vi "Main.vi"(11 "Module Admin":refnum<class "Delacor_lib_QMH_Module Admin.lvclass">) -> ()   [LabVIEW 2019, in "CONEXIÓN CON EL MICRO.lvlib"]
doc: "This template is based off of the Queued Message Handler design pattern and the Queued Message Handler project template that ships with LabVIEW.\n\nThe main difference is that the queue is private to this module and communication between modules is performed via Broadcast and Request events.\n\nRequest events are wrapped in public API methods and are handled in the Event Handling Loop (EHL) of this VI. Any module can register for Broadcast events sent by this module. The EHL generates messages based on user interface actions.\n\nThe Message Handling Loop (MHL) processes messages generated by the EHL, or by other messages. The messages are string values, so new messages can be added easily to the Message Cases case structure in the MHL. Each message cluster can also provide an optional value for Message Data, which is a variant that can be converted to whatever message-specific data is required.\n_____\nBased on Delacor QMH Project Template 5.0.0.82."
uses:
  <vilib>/Delacor/Delacor QMH/Libraries/Module Admin_class/Delacor_lib_QMH_Module Admin.lvclass
  Module Data--cluster.ctl
  <vilib>/Delacor/Delacor QMH/Libraries/Message Queue_class/Delacor_lib_QMH_Message Queue.lvclass/Delacor_lib_QMH_Message Queue.ctl
  Stop Argument--cluster.ctl
  <vilib>/Delacor/Delacor QMH/Libraries/Module Admin_class/Delacor_lib_QMH_Module Admin.lvclass/Delacor_lib_QMH_Module Admin.ctl
  START HELPER LOOP Argument--cluster.ctl
  STOP HELPER LOOP Argument--cluster.ctl
  <vilib>/Utility/miscctls.llb/LVPointTypeDef.ctl
  <vilib>/Delacor/Delacor QMH/Libraries/Message Queue_class/Delacor_lib_QMH_Enqueue Message (Single).vi
  <vilib>/Delacor/Delacor QMH/Libraries/Module Admin_class/Delacor_lib_QMH_Get External Launch.vi
  <vilib>/Utility/error.llb/Error Cluster From Error Code.vi
  <vilib>/ErrorRing/Error Ring.xnode
  <vilib>/Delacor/Delacor QMH/Libraries/Message Queue_class/Delacor_lib_QMH_Message Queue.lvclass
panel:
  in  "Simulate MHL Error":bool
  in  "Simulate EHL Error":bool
  out "error out":errorcluster
  out "Status":string
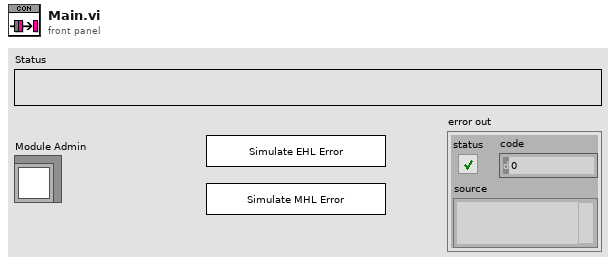
[diagram p1: front panel]
types:
  T1 = typedef "CONEXIÓN CON EL MICRO.lvlib/Request Events--cluster.ctl" = cluster{"Stop Module":refnum<user-event>, "Show Panel":refnum<user-event>, "Hide Panel":refnum<user-event>, "Get Module Execution Status":refnum<user-event>, "Show Diagram":refnum<user-event>, "START HELPER LOOP":refnum<user-event>, "STOP HELPER LOOP":refnum<user-event>}
  T2 = typedef "CONEXIÓN CON EL MICRO.lvlib/Module Data--cluster.ctl" = cluster{"Status":string}
  T3 = enum32{"invalid lock state", "Not Locked", "Locked (No Password)", "Password-protected"}
  T4 = typedef "CONEXIÓN CON EL MICRO.lvlib/Stop Argument--cluster.ctl" = cluster{"Origin":string, "Exit via Stop Module Req?":bool, "Wait for Module to stop?":bool}
  T5 = typedef "CONEXIÓN CON EL MICRO.lvlib/START HELPER LOOP Argument--cluster.ctl" = cluster{"DELAY TIMEOUT":i32}
  T6 = typedef "CONEXIÓN CON EL MICRO.lvlib/STOP HELPER LOOP Argument--cluster.ctl" = cluster{"Boolean":bool}
  T7 = typedef "LVPointTypeDef.ctl" = cluster{"Horizontal":i16, "Vertical":i16}
  T8 = enum32{"Invalid", "Standard", "Closed", "Hidden", "Minimized", "Maximized"}
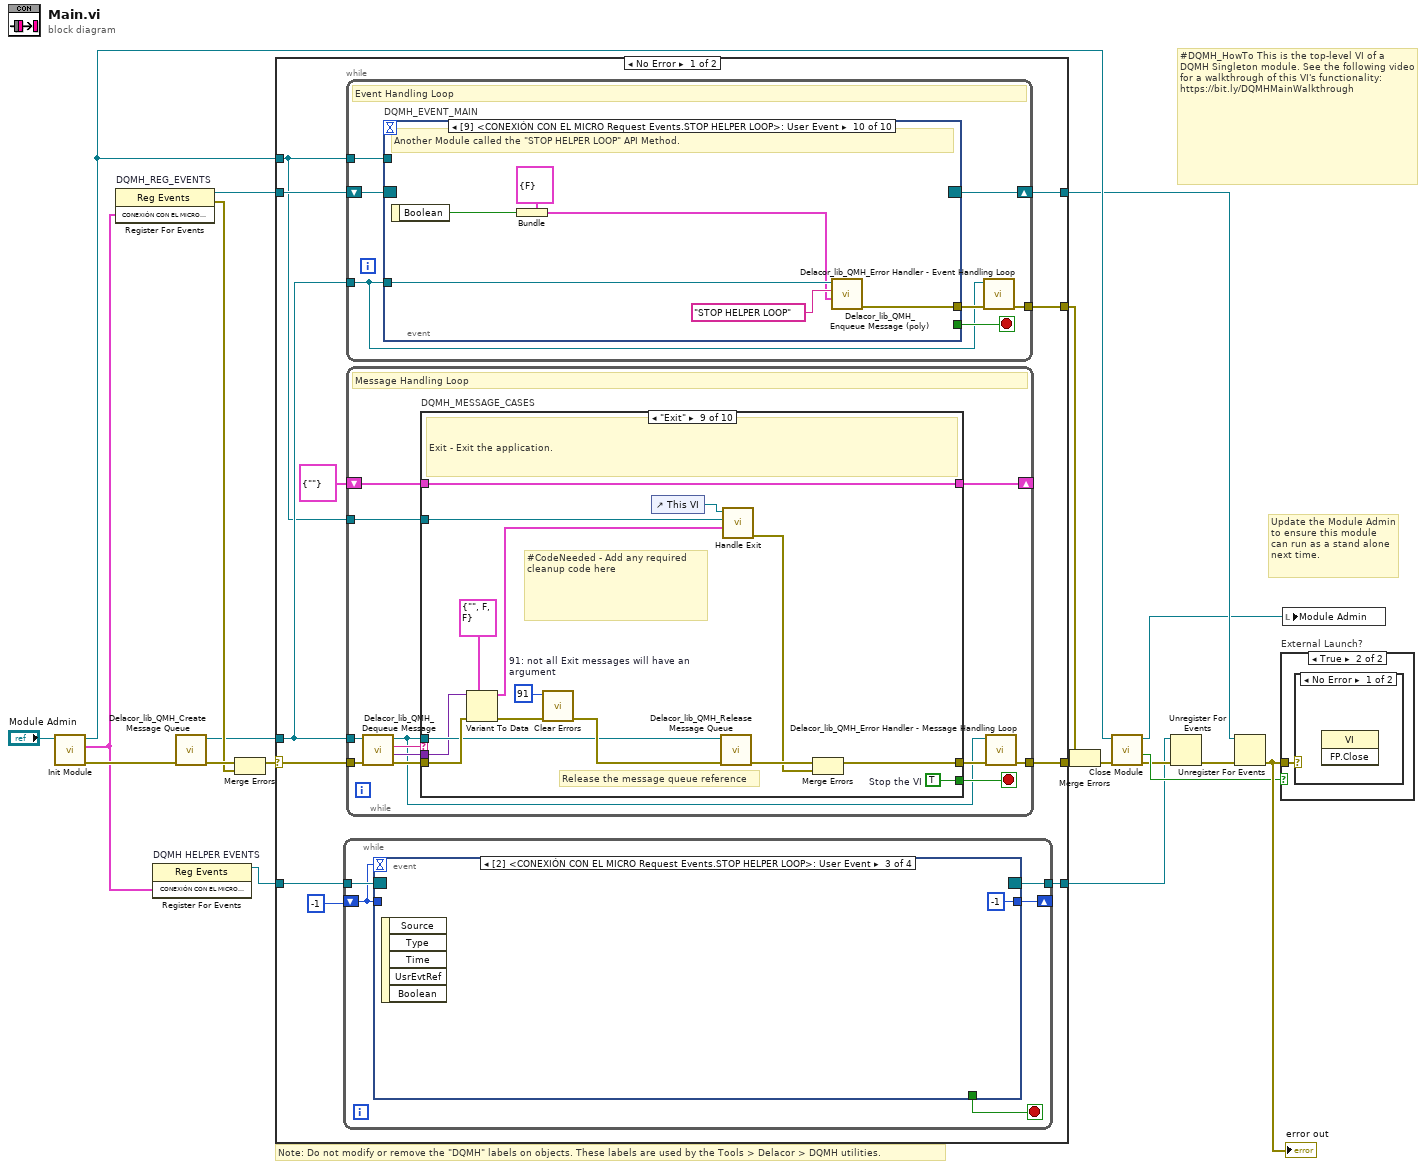
[diagram p0: block diagram]
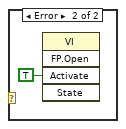
[diagram p3: hidden frame]
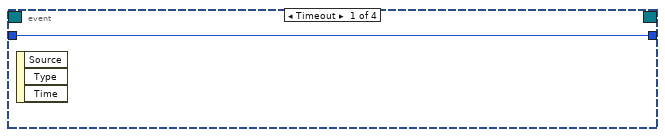
[diagram p4: hidden frame]
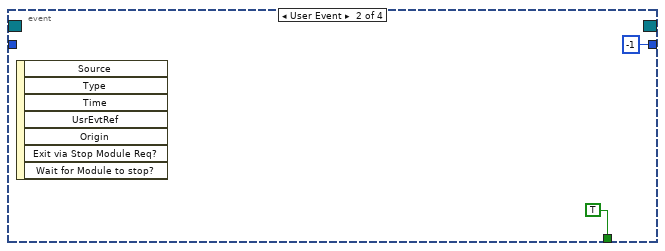
[diagram p5: hidden frame]
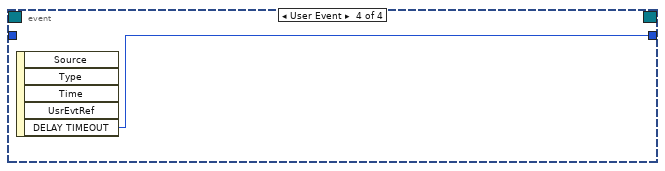
[diagram p6: hidden frame]
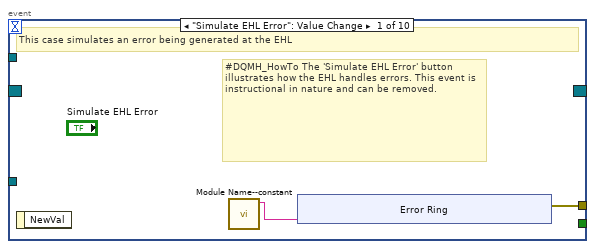
[diagram p7: hidden frame]
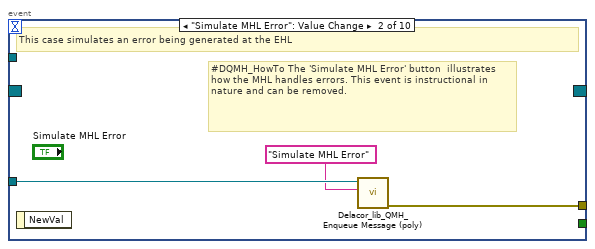
[diagram p8: hidden frame]
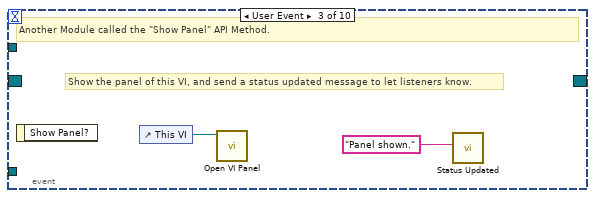
[diagram p9: hidden frame]
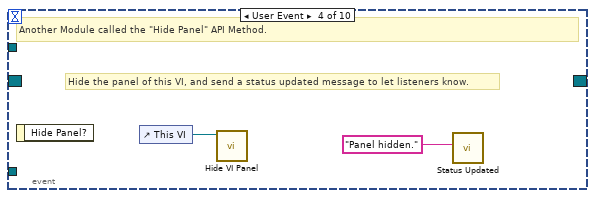
[diagram p10: hidden frame]
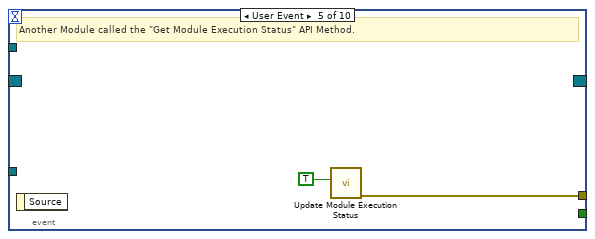
[diagram p11: hidden frame]
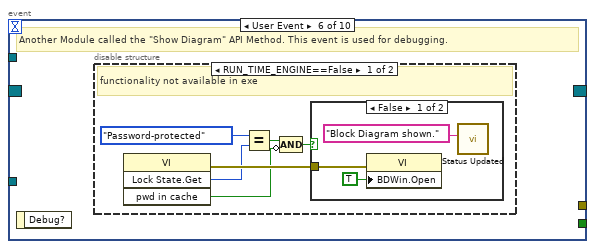
[diagram p12: hidden frame]
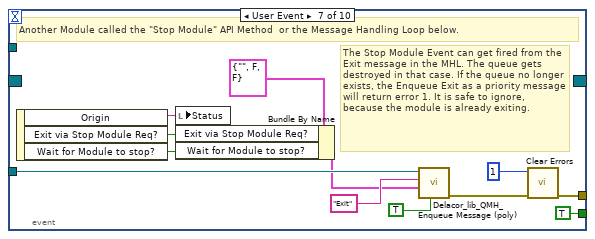
[diagram p15: hidden frame]
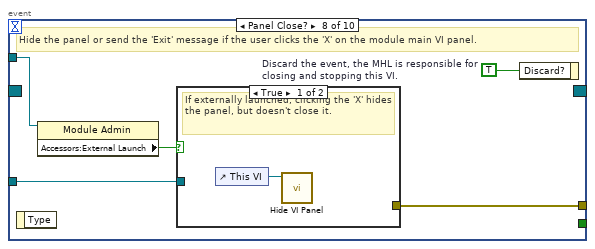
[diagram p16: hidden frame]
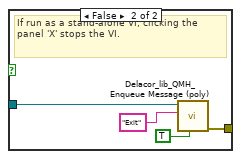
[diagram p17: hidden frame]
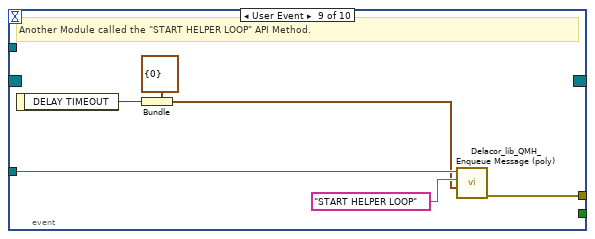
[diagram p18: hidden frame]
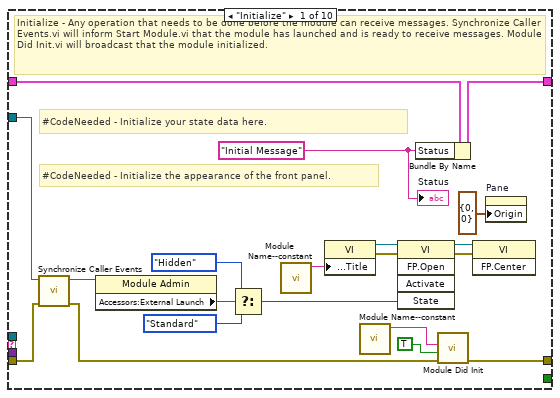
[diagram p19: hidden frame]
diagram:
  # "#DQMH_HowTo This is the top-level VI of a DQMH Singleton module. See the following video for a walkthrough of this VI's functionality: https://bit.ly/DQMHMainWalkthrough"
  # "Note: Do not modify or remove the \"DQMH\" labels on objects. These labels are used by the Tools > Delacor > DQMH utilities."
  # "Update the Module Admin to ensure this module can run as a stand alone next time."
  n1 = call "Init Module.vi"("Singleton Module Admin in"="Module Admin") -> ("error out"=w19:errorcluster, "CONEXIÓN CON EL MICRO Request Events"=w2:T1, "Singleton Module Admin out"=w12:refnum<class "Delacor_lib_QMH_Module Admin.lvclass">)  [unwired: 8 in]
  n2 = register-events "DQMH_REG_EVENTS"(w2) -> (reference out=w10:refnum<event-registration>, error out=w13:errorcluster)  [unwired: 2 in]
  n3 = register-events "DQMH HELPER EVENTS"(w2) -> (reference out=w1:refnum<event-registration>)  [unwired: 2 in, 1 out]
  n4 = call <vilib>:"Delacor_lib_QMH_Create Message Queue.vi"("error in (no error)"=w19) -> ("error out"=w15:errorcluster, "Message Queue"=w9:refnum<class "Delacor_lib_QMH_Message Queue.lvclass">)  [unwired: 9 in]
  n5 = Merge Errors(w15, w13) -> (w14:errorcluster)
  n6 = case shown="No Error" w14 {
    selector: w14 -> [w29 w222]
    tunnel: [w31 w221] -> w20
    tunnel: [w28 w227] -> w11
    tunnel: w10 -> [w26 w227]
    tunnel: w9 -> [w25 w220]
    tunnel: [w30 _] -> w18
    tunnel: w12 -> [w24 w223]
    tunnel: [w23 w219] -> w3
    tunnel: w1 -> [w22 w219]
    frame No Error {
      n7 = while {
        tunnel: [w36] -> w23
        tunnel: w22 -> [w35]
        shift-right: [w34] -> _
        shift-left: -1 -> [w33]
        stop <- w32 stop-if-true
        n8 = event shown="[2] <CONEXIÓN CON EL MICRO Request Events.STOP HELPER LOOP>: User Event" {
          selector: w35 -> [_ _ _ _]
          dyn-events: [_ _ _ _] -> w36
          timeout: w33 -> [_ _ _ _]
          tunnel: [w37 -1 ("DELAY TIMEOUT") -1 ("DELAY TIMEOUT") w41] -> w34
          tunnel: w33 -> [w37 _ _ _]
          tunnel: [_ TRUE _ _] -> w32
          event Timeout {
            n9 = event-data() -> ()  [unwired: 1 in, 3 out]
          }
          event User Event {
            n10 = event-data() -> ()  [unwired: 1 in, 7 out]
          }
          event User Event {
            n11 = event-data() -> ()  [unwired: 1 in, 5 out]
          }
          event User Event {
            n12 = event-data() -> ("DELAY TIMEOUT"=w41:i32)  [unwired: 1 in, 4 out]
          }
        }
      }
      n13 = while {
        tunnel: w25 -> [w42]
        shift-right: [w45] -> w28
        shift-left: w26 -> [w46]
        tunnel: [w47] -> w30
        tunnel: w24 -> [w43]
        stop <- w44 stop-if-true
        # "Event Handling Loop"
        n14 = event "DQMH_EVENT_MAIN" shown="[9] <CONEXIÓN CON EL MICRO Request Events.STOP HELPER LOOP>: User Event" {
          selector: w46 -> [_ _ _ _ _ _ _ _ _ _]
          dyn-events: [_ _ _ _ _ _ _ _ _ _] -> w45
          timeout: _ -> [_ _ _ _ _ _ _ _ _ _]
          tunnel: [_ _ _ _ _ _ TRUE ("Discard?") _ _ _] -> w44
          tunnel: w42 -> [_ w59 _ _ _ _ w83 w90 w103 w109]
          tunnel: [w50 w60 _ _ w66 _ w86 w92 w98 w104] -> w48
          tunnel: w43 -> [_ _ _ _ _ _ _ w89 _ _]
          event "Simulate EHL Error": Value Change {
            # "#DQMH_HowTo The 'Simulate EHL Error' button  illustrates how the EHL handles errors. This event is instructional in nature and can be removed."
            # "This case simulates an error being generated at the EHL"
            n15 = event-data() -> ()  [unwired: 1 in, 1 out]
            n16 = call "Module Name--constant.vi"() -> ("Module Name"=w49:string)  [unwired: 11 in]
            n17 = xnode "Error Ring"("parameter 0"=w49) -> ("error out"=w50:errorcluster)
          }
          event "Simulate MHL Error": Value Change {
            # "#DQMH_HowTo The 'Simulate MHL Error' button  illustrates how the MHL handles errors. This event is instructional in nature and can be removed."
            # "This case simulates an error being generated at the EHL"
            n18 = event-data() -> ()  [unwired: 1 in, 1 out]
            n19 = call-poly <vilib>:"Delacor_lib_QMH_Enqueue Message (poly).vi"("Message"="Simulate MHL Error", "Message Queue in"=w59) -> ("error out"=w60:errorcluster)  [unwired: 8 in, 1 out]
          }
          event User Event {
            # "Show the panel of this VI, and send a status updated message to let listeners know."
            # "Another Module called the \"Show Panel\" API Method."
            n20 = event-data() -> ()  [unwired: 1 in, 1 out]
            n21 = control-ref of="This VI"() -> (w62:refnum<vi>)
            n22 = call "Open VI Panel.vi"("VI"=w62) -> ()  [unwired: 10 in, 1 out]
            n23 = call "Status Updated.vi"("Status"="Panel shown." ("format string")) -> ()  [unwired: 10 in, 1 out]
          }
          event User Event {
            # "Hide the panel of this VI, and send a status updated message to let listeners know."
            # "Another Module called the \"Hide Panel\" API Method."
            n24 = event-data() -> ()  [unwired: 1 in, 1 out]
            n25 = control-ref of="This VI"() -> (w64:refnum<vi>)
            n26 = call "Hide VI Panel.vi"("VI"=w64) -> ()  [unwired: 10 in, 1 out]
            n27 = call "Status Updated.vi"("Status"="Panel hidden." ("format string")) -> ()  [unwired: 10 in, 1 out]
          }
          event User Event {
            # "Another Module called the \"Get Module Execution Status\" API Method."
            n28 = event-data() -> ()  [unwired: 1 in, 1 out]
            n29 = call "Update Module Execution Status.vi"("Running?"=TRUE) -> ("error out"=w66:errorcluster)  [unwired: 10 in]
          }
          event User Event {
            # "Another Module called the \"Show Diagram\" API Method. This event is used for debugging."
            n30 = event-data() -> ()  [unwired: 1 in, 1 out]
            n31 = disable-structure shown="RUN_TIME_ENGINE==False" {
              frame condition #0 (active) {
                # "functionality not available in exe"
                n32 = invoke class="VI" method="Lock State.Get"() -> (error out=w72:errorcluster, "Get Lock State"=w71:T3, "pwd in cache"=w68:bool)  [unwired: 4 in, 1 out]
                n33 = Equal?(x=T3."Password-protected", y=w71) -> (x = y?=w69:bool)
                n34 = Compound Arithmetic op=AND(w69, invert w68) -> (w67:bool)
                n35 = case shown="False" w67 {
                  tunnel: w72 -> [w75 _]
                  frame False {
                    n36 = property class="VI"(error in=w75, "BDWin.Open"=TRUE ("Block Diagram Window:Open")) -> ()  [unwired: 1 in, 2 out]
                    n37 = call "Status Updated.vi"("Status"="Block Diagram shown." ("format string")) -> ()  [unwired: 10 in, 1 out]
                  }
                  frame True {
                    # "Password-protected VI, and the password is not in the cache. Do not show the diagram."
                  }
                }
              }
              frame condition #1 {
              }
            }
          }
          event User Event {
            # "The Stop Module Event can get fired from the Exit message in the MHL. The queue gets destroyed in that case. If the queue no longer exists, the Enqueue Exit as a priority message will return error 1. It is safe to ignore, because the module is already exiting."
            # "Another Module called the \"Stop Module\" API Method  or the Message Handling Loop below."
            n38 = event-data() -> ("Origin"=w82:string, "Exit via Stop Module Req?"=w78:bool, "Wait for Module to stop?"=w77:bool)  [unwired: 1 in]
            n39 = local write "Status"(w82) -> ()
            n40 = Bundle By Name(cluster=T4 {"Origin"="", "Exit via Stop Module Req?"=FALSE, "Wait for Module to stop?"=FALSE} ("Stop Argument"), "Exit via Stop Module Req?"=w78, "Wait for Module to stop?"=w77) -> (w76:T4)
            n41 = call-poly <vilib>:"Delacor_lib_QMH_Enqueue Message (poly).vi"("Priority Message? (F)"=TRUE, "Message Data"=w76, "Message"="Exit", "Message Queue in"=w83) -> ("error out"=w87:errorcluster)  [unwired: 6 in, 1 out]
            n42 = call <vilib>:"Clear Errors.vi"("error in (no error)"=w87, "specific error code to clear (0: all)"=1) -> ("error out"=w86:errorcluster)  [unwired: 4 in, 1 out]
          }
          event Panel Close? {
            w91 = TRUE  # Discard the event, the MHL is responsible for closing and stopping this VI.
            # "Hide the panel or send the 'Exit' message if the user clicks the 'X' on the module main VI panel."
            n43 = event-data() -> ()  [unwired: 1 in, 1 out]
            n44 = property class="Module Admin"(reference=w89) -> ("Accessors:External Launch"=w88:bool)  [unwired: 1 in, 2 out]
            n45 = case shown="True" w88 {
              tunnel: w90 -> [_ w96]
              tunnel: [_ w97] -> w92
              frame True {
                # "If externally launched, clicking the 'X' hides the panel, but doesn't close it."
                n46 = control-ref of="This VI"() -> (w93:refnum<vi>)
                n47 = call "Hide VI Panel.vi"("VI"=w93) -> ()  [unwired: 10 in, 1 out]
              }
              frame False {
                # "If run as a stand-alone VI, clicking the panel 'X' stops the VI."
                n48 = call-poly <vilib>:"Delacor_lib_QMH_Enqueue Message (poly).vi"("Priority Message? (F)"=TRUE, "Message"="Exit", "Message Queue in"=w96) -> ("error out"=w97:errorcluster)  [unwired: 7 in, 1 out]
              }
            }
            n49 = event-data("Discard?"=w91) -> ()  [unwired: 1 in, 1 out]
          }
          event User Event {
            # "Another Module called the \"START HELPER LOOP\" API Method."
            n50 = event-data() -> ("DELAY TIMEOUT"=w99:i32)  [unwired: 1 in]
            n51 = Bundle(cluster=T5 {"DELAY TIMEOUT"=0} ("START HELPER LOOP Argument"), "DELAY TIMEOUT"=w99) -> (w100:T5)
            n52 = call-poly <vilib>:"Delacor_lib_QMH_Enqueue Message (poly).vi"("Message Data"=w100, "Message"="START HELPER LOOP", "Message Queue in"=w103) -> ("error out"=w98:errorcluster)  [unwired: 7 in, 1 out]
          }
          event User Event {
            # "Another Module called the \"STOP HELPER LOOP\" API Method."
            n53 = event-data() -> ("Boolean"=w105:bool)  [unwired: 1 in]
            n54 = Bundle(cluster=T6 {"Boolean"=FALSE} ("STOP HELPER LOOP Argument"), "Boolean"=w105) -> (w106:T6)
            n55 = call-poly <vilib>:"Delacor_lib_QMH_Enqueue Message (poly).vi"("Message Data"=w106, "Message"="STOP HELPER LOOP", "Message Queue in"=w109) -> ("error out"=w104:errorcluster)  [unwired: 7 in, 1 out]
          }
        }
        n56 = call-dynamic "Delacor_lib_QMH_Error Handler - Event Handling Loop.vi"("error in (no error)"=w48, "Message Queue in"=w42) -> ("dup error in"=w47:errorcluster)  [unwired: 8 in, 1 out]
      }
      n57 = while {
        tunnel: w25 -> [w112]
        shift-right: [w116] -> _
        shift-left: T2 {"Status"=""} ("Data Cluster") -> [w117]
        tunnel: w29 -> [w120]
        tunnel: [w118] -> w31
        tunnel: w24 -> [w110]
        stop <- w115 stop-if-true
        # "Message Handling Loop"
        n58 = call-dynamic "Delacor_lib_QMH_Dequeue Message.vi"("error in (no error)"=w120, "Message Queue in"=w112) -> ("error out"=w119:errorcluster, "Message Data"=w113:variant, "Message"=w114:string, "Message Queue out"=w111:refnum<class "Delacor_lib_QMH_Message Queue.lvclass">)  [unwired: 6 in]
        n59 = case "DQMH_MESSAGE_CASES" shown="\"Exit\"" w114 {
          selector: w114 -> [_ _ _ _ _ _ _ _ _ w206]
          tunnel: w111 -> [_ _ _ _ _ _ _ w176 w198 _]
          tunnel: w119 -> [w139 w143 w149 w155 w158 w160 w165 w183 w204 w208]
          tunnel: [w137 w143 w147 w153 w157 w160 w164 w179 w201 w209] -> w121
          tunnel: w117 -> [w128 w142 w148 w154 w156 w159 w162 w178 w197 w207]
          tunnel: [w127 w142 w148 w154 w156 w159 w162 w178 w197 w207] -> w116
          tunnel: [_ _ _ _ _ _ _ _ w196 _] -> w115
          tunnel: w113 -> [_ _ w146 w152 _ _ _ w177 w195 _]
          tunnel: w110 -> [w129 _ _ _ _ _ _ w175 w190 _]
          frame "Initialize" {
            w122 = "Initial Message" ("Initial Message")
            # "#CodeNeeded - Initialize the appearance of the front panel."
            # "#CodeNeeded - Initialize your state data here."
            # "Initialize - Any operation that needs to be done before the module can receive messages. Synchronize Caller Events.vi will inform Start Module.vi that the module has launched and is ready to receive messages. Module Did Init.vi will broadcast that the module initialized."
            n60 = call "Synchronize Caller Events.vi"("error in (no error)"=w139, "Singleton Module Admin in"=w129) -> ("error out"=w138:errorcluster, "Singleton Module Admin out"=w124:refnum<class "Delacor_lib_QMH_Module Admin.lvclass">)  [unwired: 8 in]
            n61 = property class="Module Admin"(reference=w124) -> ("Accessors:External Launch"=w133:bool)  [unwired: 1 in, 2 out]
            n62 = Select(t=T8."Hidden" ("State"), s=w133, f=T8."Standard" ("State")) -> (s? t:f=w130:T8)
            n63 = call "Module Name--constant.vi"() -> ("Module Name"=w136:string)  [unwired: 11 in]
            n64 = property class="VI"("Front Panel.Title"=w136) -> (reference out=w135:refnum<vi>, error out=w141:errorcluster)  [unwired: 2 in]
            n65 = call "Module Name--constant.vi"() -> ("Module Name"=w125:string)  [unwired: 11 in]
            n66 = invoke class="VI" method="FP.Open"(reference=w135, error in=w141, "State"=w130) -> (reference out=w134:refnum<vi>, error out=w140:errorcluster)  [unwired: 2 in, 3 out]
            n67 = Bundle By Name(cluster=w128, "Status"=w122) -> (w127:T2)
            n68 = call "Module Did Init.vi"("error in (no error)"=w138, "Initialized?"=TRUE, "Origin"=w125) -> ("error out"=w137:errorcluster)  [unwired: 8 in]
            n69 = invoke class="VI" method="FP.Center"(reference=w134, error in=w140) -> ()  [unwired: 1 in, 3 out]
            n70 = property on="Pane" class="Pane"("Origin"=T7 {"Horizontal"=0, "Vertical"=0}) -> ()  [unwired: 2 in, 2 out]
            "Status" <- w122
          }
          frame "--- Module Specific ---" {
            # "Separator -- The following cases handle messages specific to this Module."
          }
          frame "START HELPER LOOP" {
            # "#CodeNeeded\n1. Configure this Message Case for handling the \"START HELPER LOOP\" message.\n2. Delete or edit this label when done."
            # "INICIALIZAR HELPER LOOP"
            n71 = Variant To Data(error in=w149, type=T5 {"DELAY TIMEOUT"=0} ("START HELPER LOOP Argument"), Variant=w146) -> (data=w144:T5, error out=w147:errorcluster)
            n72 = Unbundle By Name(w144) -> ()  [unwired: 1 out]
          }
          frame "STOP HELPER LOOP" {
            # "#CodeNeeded\n1. Configure this Message Case for handling the \"STOP HELPER LOOP\" message.\n2. Delete or edit this label when done."
            # "STOP HELPER LOOP"
            n73 = Variant To Data(error in=w155, type=T6 {"Boolean"=FALSE} ("STOP HELPER LOOP Argument"), Variant=w152) -> (data=w150:T6, error out=w153:errorcluster)
            n74 = Unbundle By Name(w150) -> ()  [unwired: 1 out]
          }
          frame "---Copy This Frame---" {
            # "Duplicate this frame when creating new messages.  Change this comment in the duplicated frame to describe this message."
            n75 = Merge Errors(w158) -> (w157:errorcluster)
          }
          frame "--- Exit and Error Handling---" {
            # "Separator - The following cases handle errors and exit messages."
          }
          frame "Simulate MHL Error" {
            # "#DQMH_HowTo The 'Simulate MHL Error' button  illustrates how the MHL handles errors. This event is instructional in nature and can be removed."
            # "Simulate an error occurring at the MHL"
            n76 = call "Module Name--constant.vi"() -> ("Module Name"=w161:string)  [unwired: 11 in]
            n77 = xnode "Error Ring"("parameter 0"=w161) -> ("error out"=w163:errorcluster)
            n78 = Merge Errors(w165, w163) -> (w164:errorcluster)
          }
          frame "Error" {
            # "#CodeRecommended - If you ever change the name of this \"Error\" message, you'll need to update the name in the Check Loop Error.vi as well."
            # "#CodeRecommended - If the module is running in standalone mode (External Launch = FALSE), this code will pop up an error dialog and call the 'Exit' message if an error occurs. Add more fine-grained error handling here."
            # "Error - Check the error message data and respond accordingly. This message is sent by the \"Error Handler\" VIs at the end of each loop in this application."
            n79 = property class="Module Admin"(reference=w175) -> ("Accessors:External Launch"=w174:bool)  [unwired: 1 in, 2 out]
            n80 = Variant To Data(error in=w183, type=errorcluster {"status"=FALSE, "code"=0, "source"=""} ("error constant"), Variant=w177) -> (data=w184:errorcluster, error out=w181:errorcluster)
            n81 = call "Module Name--constant.vi"() -> ("Module Name"=w173:string)  [unwired: 11 in]
            n82 = call "Error Reported.vi"("Additional Information"=w173, "Error"=w184) -> ()  [unwired: 9 in, 1 out]
            n83 = case shown="False" w174 {
              tunnel: [w189 _] -> w180
              tunnel: w176 -> [w187 _]
              tunnel: w184 -> [w188 _]
              frame False {
                # "If the module is running standalone, then pop up an error dialog and call the \"Exit\" message."
                n84 = call <vilib>:"Simple Error Handler.vi"("error in (no error)"=w188) -> ()  [unwired: 4 in, 5 out]
                n85 = call-poly <vilib>:"Delacor_lib_QMH_Enqueue Message (poly).vi"("Priority Message? (F)"=TRUE, "Message"="Exit", "Message Queue in"=w187) -> ("error out"=w189:errorcluster)  [unwired: 7 in, 1 out]
              }
              frame True {
                # "If the module was launched externally, calling the Error Reported broadcast VI is the only action performed by the \"Error\" message. The module's caller can then process the error appropriately."
              }
            }
            n86 = Merge Errors(w181, w180) -> (w179:errorcluster)
            n87 = local write "error out"(w179) -> ()
          }
          frame "Exit" {
            w194 = 91  # 91: not all Exit messages will have an argument
            w196 = TRUE  # Stop the VI
            # "Release the message queue reference"
            # "#CodeNeeded - Add any required cleanup code here"
            # "Exit - Exit the application."
            n88 = Variant To Data(error in=w204, type=T4 {"Origin"="", "Exit via Stop Module Req?"=FALSE, "Wait for Module to stop?"=FALSE} ("Stop Argument"), Variant=w195) -> (data=w192:T4, error out=w200:errorcluster)
            n89 = call <vilib>:"Clear Errors.vi"("error in (no error)"=w200, "specific error code to clear (0: all)"=w194) -> ("error out"=w203:errorcluster)  [unwired: 4 in, 1 out]
            n90 = control-ref of="This VI"() -> (w191:refnum<vi>)
            n91 = call-dynamic "Delacor_lib_QMH_Release Message Queue.vi"("error in (no error)"=w203, "Message Queue"=w198) -> ("error out"=w202:errorcluster)  [unwired: 9 in]
            n92 = call "Handle Exit.vi"("Stop Argument"=w192, "Admin in"=w190, "VI reference"=w191) -> ("error out"=w199:errorcluster)  [unwired: 7 in, 1 out]
            n93 = Merge Errors(w202, w199) -> (w201:errorcluster)
          }
          frame Default {
            # "'Default' case only runs if there is a message that isn't defined in any of the other cases.  Output a programming error."
            n94 = call "Module Name--constant.vi"() -> ("Module Name"=w205:string)  [unwired: 11 in]
            n95 = xnode "Error Ring"("parameter 0"=w206, "parameter 1"=w205) -> ("error out"=w210:errorcluster)
            n96 = Merge Errors(w208, w210) -> (w209:errorcluster)
          }
        }
        n97 = call-dynamic "Delacor_lib_QMH_Error Handler - Message Handling Loop.vi"("error in (no error)"=w121, "Message Queue in"=w111) -> ("dup error in"=w118:errorcluster)  [unwired: 8 in, 1 out]
      }
    }
    frame Error {
      # "Synchronize Caller Events.vi will inform Start Module.vi that the module has launched and will let the code calling Start Module.vi register for broadcasts and would permit the caller receive the broadcast that an error occurred at launch time."
      n98 = call-dynamic "Delacor_lib_QMH_Release Message Queue.vi"("error in (no error)"=w222, "Message Queue"=w220) -> ("error out"=w221:errorcluster)  [unwired: 9 in]
      n99 = call "Synchronize Caller Events.vi"("Singleton Module Admin in"=w223) -> ("error out"=w228:errorcluster)  [unwired: 9 in, 1 out]
      n100 = call "Module Name--constant.vi"() -> ("Module Name"=w226:string)  [unwired: 11 in]
      n101 = Format Into String(format string="An error occurred during initialization. %s is no longer running.", w226) -> (resulting string=w224:string)  [unwired: 2 in, 1 out]
      n102 = Merge Errors(w221, w228) -> (w229:errorcluster)
      n103 = call "Error Reported.vi"("Additional Information"=w224, "Error"=w229) -> ()  [unwired: 9 in, 1 out]
    }
  }
  n104 = Merge Errors(w18, w20) -> (w17:errorcluster)
  n105 = call "Close Module.vi"("error in (no error)"=w17, "Module Admin in"=w12) -> ("error out"=w4:errorcluster, "External Launch"=w6:bool, "Module Admin out"=w7:refnum<class "Delacor_lib_QMH_Module Admin.lvclass">)  [unwired: 7 in]
  n106 = Unregister For Events(event registration refnum=w3, error in=w4) -> (error out=w5:errorcluster)
  n107 = Unregister For Events(event registration refnum=w11, error in=w5) -> (error out=w16:errorcluster)
  "error out" <- w16
  n108 = case "External Launch?" shown="True" w6 {
    tunnel: w16 -> [_ w230]
    frame False {
    }
    frame True {
      n109 = case shown="No Error" w230 {
        frame No Error {
          n110 = invoke class="VI" method="FP.Close"() -> ()  [unwired: 3 in, 3 out]
        }
        frame Error {
          n111 = invoke class="VI" method="FP.Open"("Activate"=TRUE ("Activate?")) -> ()  [unwired: 4 in, 5 out]
        }
      }
    }
  }
  n112 = local write "Module Admin"(w7) -> ()
